vi "探头修改系数指令.vi"(9 "N2":u16, 10 "N1":u16, 11 "探头地址":u8) -> (3 "改系数指令":string)   [LabVIEW 2017]
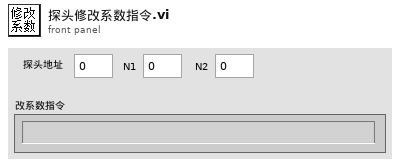
[diagram p1: front panel]
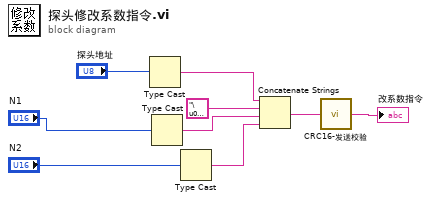
[diagram p0: block diagram]
diagram:
  n1 = Type Cast(x="探头地址") -> (*(type *) &x=w2:string)  [unwired: 1 in]
  n2 = Type Cast(x="N1") -> (*(type *) &x=w7:string)  [unwired: 1 in]
  n3 = Type Cast(x="N2") -> (*(type *) &x=w5:string)  [unwired: 1 in]
  n4 = Concatenate Strings(w2, "\u0012", w7, w5) -> (w4:string)
  n5 = call "CRC16-发送校验.vi"("净数据"=w4) -> ("完整输出"=→"改系数指令":string)
